vi "Number Pad.vi"(0 "Instruction":string="Please Enter Setpoint", 7 "CtlRef":refnum<vi>, 9 "Array Element":refnum<vi>, 11 "Error Input":errorcluster) -> (4 "String":string="0", 8 "Numeric":dbl=32.0, 15 "Error Output":errorcluster)   [LabVIEW 2010]
panel:
  out "Text Description":string="Please Enter Setpoint"
  in  "Cancel":bool
  in  "dot":bool
  in  "0":bool
  in  "9":bool
  in  "8":bool
  in  "7":bool
  in  "6":bool
  in  "5":bool
  in  "4":bool
  in  "3":bool
  in  "2":bool
  in  "1":bool
  in  "clear":bool
  in  "Backspace":bool
  in  "OK":bool
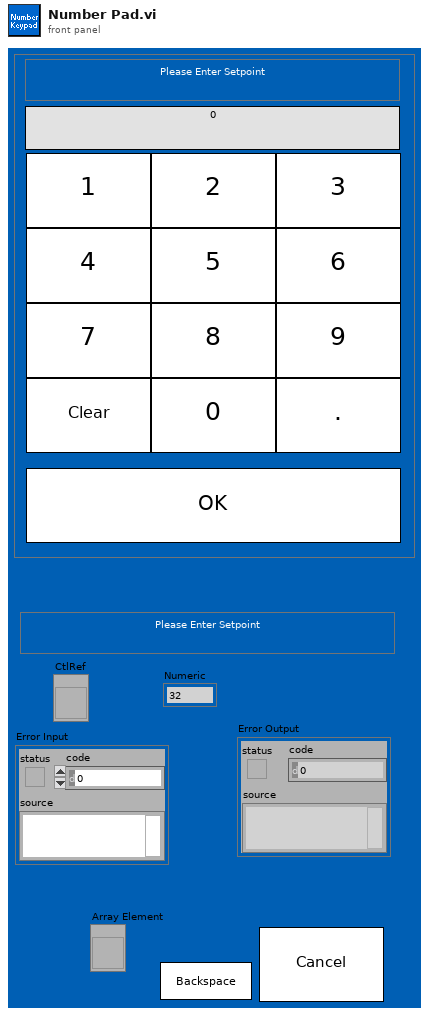
[diagram p1: front panel]
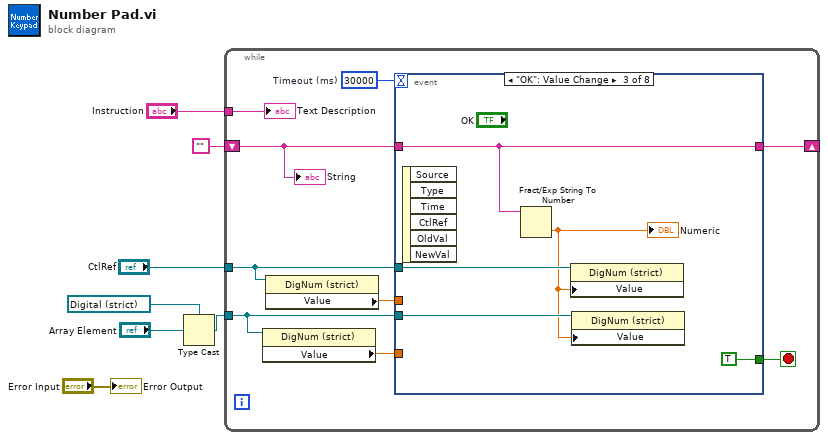
[diagram p0: block diagram]
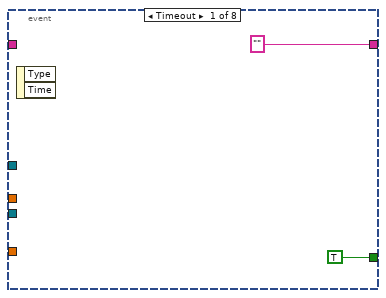
[diagram p2: hidden frame]
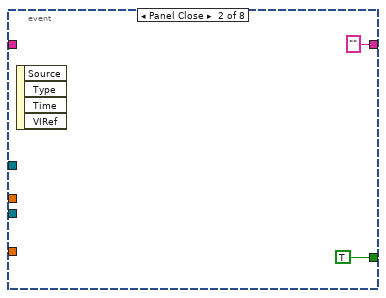
[diagram p3: hidden frame]
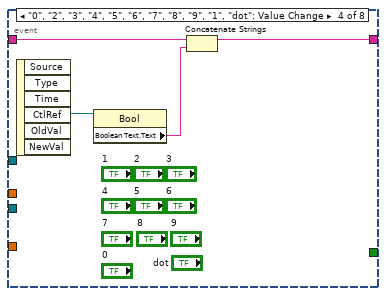
[diagram p4: hidden frame]
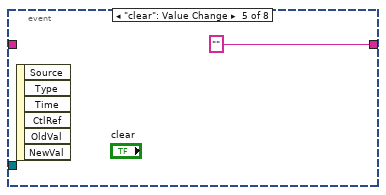
[diagram p5: hidden frame]
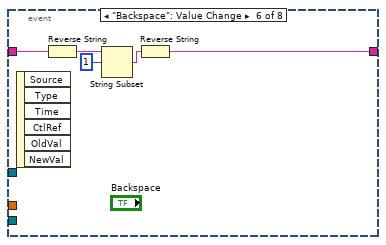
[diagram p6: hidden frame]
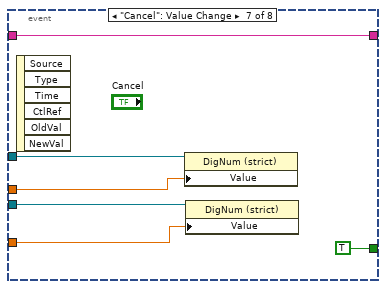
[diagram p7: hidden frame]
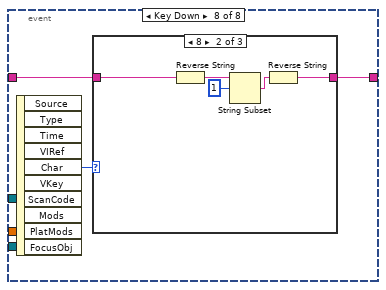
[diagram p8: hidden frame]
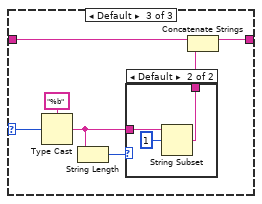
[diagram p10: hidden frame]
diagram:
  n1 = Type Cast(type=refnum<vi> refnum ("CtlRef 2"), x="Array Element") -> (*(type *) &x=w3:refnum<vi>)
  n2 = while {
    shift-right: [w16] -> _
    shift-left: "" -> [w9]
    tunnel: "CtlRef" -> [w14]
    tunnel: w3 -> [w13]
    tunnel: "Instruction" -> [w8]
    stop <- w15 stop-if-true
    w10 = 30000  # Timeout (ms)
    n3 = property class="DigNum (strict)"(reference=w13) -> ("Value"=w11:dbl)  [unwired: 1 in, 2 out]
    n4 = property class="DigNum (strict)"(reference=w14) -> ("Value"=w12:dbl)  [unwired: 1 in, 2 out]
    n5 = event shown="[2] \"OK\": Value Change" {
      selector: _ -> [_ _ _ _ _ _ _ _]
      dyn-events: _ -> [_ _ _ _ _ _ _ _]
      timeout: w10 -> [_ _ _ _ _ _ _ _]
      tunnel: [TRUE TRUE ("OK") TRUE ("OK") _ _ _ TRUE ("OK") _] -> w15
      tunnel: w9 -> [_ _ w24 w27 _ w35 w41 w44]
      tunnel: ["" "" w24 w28 "" w31 w41 w43] -> w16
      tunnel: w14 -> [_ _ w23 _ _ _ w37 _]
      tunnel: w13 -> [_ _ w22 _ _ _ w36 _]
      tunnel: w12 -> [_ _ _ _ _ _ w39 _]
      tunnel: w11 -> [_ _ _ _ _ _ w38 _]
      event Timeout {
        n6 = event-data() -> ()  [unwired: 3 out]
      }
      event Panel Close {
        n7 = event-data() -> ()  [unwired: 5 out]
      }
      event "OK": Value Change {
        n8 = event-data() -> ()  [unwired: 7 out]
        n9 = Fract/Exp String To Number(string=w24) -> (number=w21:dbl)  [unwired: 4 out]
        "Numeric" <- w21
        n10 = property class="DigNum (strict)"(reference=w23, "Value"=w21) -> ()  [unwired: 1 in, 2 out]
        n11 = property class="DigNum (strict)"(reference=w22, "Value"=w21) -> ()  [unwired: 1 in, 2 out]
      }
      event "0", "2", "3", "4", "5", "6", "7", "8", "9", "1", "dot": Value Change {
        n12 = event-data() -> ("CtlRef"=w29:refnum<vi>)  [unwired: 6 out]
        n13 = property class="Bool"(reference=w29) -> ("Boolean Text.Text"=w26:string)  [unwired: 1 in, 2 out]
        n14 = Concatenate Strings(w27, w26) -> (w28:string)
      }
      event "clear": Value Change {
        n15 = event-data() -> ()  [unwired: 7 out]
      }
      event "Backspace": Value Change {
        n16 = event-data() -> ()  [unwired: 7 out]
        n17 = Reverse String(1:w35) -> (0:w34:string)
        n18 = String Subset(string=w34, offset (0)=1) -> (substring=w32:string)  [unwired: 1 out]
        n19 = Reverse String(1:w32) -> (0:w31:string)
      }
      event "Cancel": Value Change {
        n20 = event-data() -> ()  [unwired: 7 out]
        n21 = property class="DigNum (strict)"(reference=w37, "Value"=w39) -> ()  [unwired: 1 in, 2 out]
        n22 = property class="DigNum (strict)"(reference=w36, "Value"=w38) -> ()  [unwired: 1 in, 2 out]
      }
      event Key Down {
        n23 = event-data() -> ("Char"=w42:i16)  [unwired: 10 out]
        n24 = case shown="8" w42 {
          selector: w42 -> [_ _ w54]
          tunnel: w44 -> [w45 w47 w56]
          tunnel: [w45 w46 w55] -> w43
          frame 0 {
            # "Shift key was pressed\nOmit it."
          }
          frame 8 {
            n25 = Reverse String(1:w47) -> (0:w50:string)
            n26 = String Subset(string=w50, offset (0)=1) -> (substring=w48:string)  [unwired: 1 out]
            n27 = Reverse String(1:w48) -> (0:w46:string)
          }
          frame Default {
            n28 = Type Cast(type="%b", x=w54) -> (*(type *) &x=w53:string)
            n29 = String Length(string=w53) -> (length=w51:i32)
            n30 = case shown="Default" w51 {
              tunnel: w53 -> [w58 w61]
              tunnel: [w58 w60] -> w52
              frame ..1 {
              }
              frame Default {
                n31 = String Subset(string=w61, offset (0)=1) -> (substring=w60:string)  [unwired: 1 out]
              }
            }
            n32 = Concatenate Strings(w56, w52) -> (w55:string)
          }
        }
      }
    }
    "String" <- w9
    "Text Description" <- w8
  }
  "Error Output" <- "Error Input"
